vi "诊断标定3 - 副本.vi"(8 "CAN端口":u16(ring), 9 "设备索引号":u16(ring), 10 "CAN卡类型":u32(ring)=21) -> ()   [LabVIEW 2013] (continued)
                                n3186 = Reverse 1D Array(array=w4302) -> (reversed array=w4301:i32[])
                                n3187 = for {
                                N: w4297 -> [_]
                                tunnel: w4301 -> [w4319] mode=indexing
                                tunnel: [w4315] -> w4299 mode=indexing
                                n3188 = Equal To 0?(x=w4319) -> (x = 0?=w4318:bool)
                                n3189 = Select(t="无", s=w4318, f="故障") -> (s? t:f=w4315:string)
                                }
                                n3190 = Insert Into Array(array=w4300, new element=w4299) -> (w4298:string[])  [unwired: 1 in]
                              }
                              n3191 = call "详细故障分解.vi"("名称"=string[] ["自检异常(ee_cpu)", "存储空间满(ee_cpu)", "数据写入失败(ee_cpu)", "数据读取异常(ee_cpu)", "自检异常(ee_ext)", "存储空间满(ee_ext)", "数据写入失败(ee_ext)", "数据读取异常(ee_ext)", "自检异常(flash_ext)", "故障数据存储空间满(flash_ext)", "历史数据存储空间满(flash_ext)", "数据写入失败(flash_ext)", "数据读取失败(flash_ext)", "数据校验异常(flash_ext)", "自检异常(flash_cpu)", "存储空间满(flash_cpu)", "数据写入失败(flash_cpu)", "数据读取异常(flash_cpu)", "应用程序异常(cpu)", "应用程序下载异常(cpu)", "AD模块异常(cpu)", "RAM异常(cpu)", "CPU异常下电(cpu)"], "故障输入口"=w4292) -> ("输出数组"=w4290:string[][])  [unwired: 1 in, 2 out]
                              n3192 = local write "电池故障"(w4290) -> ()
                            }
                            frame 3 {
                              n3193 = for {
                                N: 5 -> [_]
                                tunnel: w4324 -> [w4341]
                                shift-right: [w4328] -> w4322
                                shift-left: string[] [] -> [w4330]
                                i -> [w4327]
                                w4335 = 8 ("索引")
                                w4339 = 2 ("y")
                                n3194 = Multiply(x=w4327, y=w4339) -> (x*y=w4340:i32)
                                n3195 = Array Subset(array=w4341, index=w4340, length=w4339) -> (w4338:u8[])
                                n3196 = Index Array(array=w4338) -> (element #1=w4337:u8, element #2=w4336:u8)  [unwired: 2 in]
                                n3197 = call "二进制解析-8.6.vi"("索引"=w4335, "数值"=w4337) -> ("低位子数组"=w4334:i32[])  [unwired: 1 in, 2 out]
                                n3198 = call "二进制解析-8.6.vi"("索引"=w4335, "数值"=w4336) -> ("低位子数组"=w4333:i32[])  [unwired: 1 in, 2 out]
                                n3199 = Insert Into Array(array=w4334, new element=w4333) -> (w4332:i32[])  [unwired: 1 in]
                                n3200 = Reverse 1D Array(array=w4332) -> (reversed array=w4331:i32[])
                                n3201 = for {
                                N: 6 -> [_]
                                tunnel: w4331 -> [w4346] mode=indexing
                                tunnel: [w4342] -> w4329 mode=indexing
                                n3202 = Equal To 0?(x=w4346) -> (x = 0?=w4345:bool)
                                n3203 = Select(t="无", s=w4345, f="故障") -> (s? t:f=w4342:string)
                                }
                                n3204 = Insert Into Array(array=w4330, new element=w4329) -> (w4328:string[])  [unwired: 1 in]
                              }
                              n3205 = call "详细故障分解.vi"("名称"=string[] ["初始化失败(CAN4)", "发送异常(CAN4)", "接收异常(CAN4)", "总线超时(CAN4)", "BUSOFF(CAN4)", "帧格式(CAN4)", "初始化异常(CAN0)", "发送异常(CAN0)", "接收异常(CAN0)", "总线超时(CAN0)", "BUSOFF(CAN0)", "帧格式(CAN0)", "初始化异常(CAN1)", "发送异常(CAN1)", "接收异常(CAN1)", "总线超时(CAN1)", "BUSOFF(CAN1)", "帧格式(CAN1)", "初始化失败(CAN2)", "发送异常(CAN2)", "接收异常(CAN2)", "总线超时(CAN2)", "BUSOFF(CAN2)", "帧格式(CAN2)", "初始化失败(CAN3)", "发送异常(CAN3)", "接收异常(CAN3)", "总线超时(CAN3)", "BUSOFF(CAN3)", "帧格式(CAN3)"], "故障输入口"=w4322) -> ("输出数组"=w4320:string[][])  [unwired: 1 in, 2 out]
                              n3206 = local write "电池故障"(w4320) -> ()
                            }
                            frame 4 {
                              n3207 = for {
                                N: 1 -> [_]
                                tunnel: w4351 -> [w4368]
                                shift-right: [w4355] -> w4349
                                shift-left: string[] [] -> [w4357]
                                i -> [w4354]
                                w4362 = 8 ("索引")
                                w4366 = 2 ("y")
                                n3208 = Multiply(x=w4354, y=w4366) -> (x*y=w4367:i32)
                                n3209 = Array Subset(array=w4368, index=w4367, length=w4366) -> (w4365:u8[])
                                n3210 = Index Array(array=w4365) -> (element #1=w4364:u8, element #2=w4363:u8)  [unwired: 2 in]
                                n3211 = call "二进制解析-8.6.vi"("索引"=w4362, "数值"=w4364) -> ("低位子数组"=w4361:i32[])  [unwired: 1 in, 2 out]
                                n3212 = call "二进制解析-8.6.vi"("索引"=w4362, "数值"=w4363) -> ("低位子数组"=w4360:i32[])  [unwired: 1 in, 2 out]
                                n3213 = Insert Into Array(array=w4361, new element=w4360) -> (w4359:i32[])  [unwired: 1 in]
                                n3214 = Reverse 1D Array(array=w4359) -> (reversed array=w4358:i32[])
                                n3215 = for {
                                N: 4 -> [_]
                                tunnel: w4358 -> [w4373] mode=indexing
                                tunnel: [w4369] -> w4356 mode=indexing
                                n3216 = Equal To 0?(x=w4373) -> (x = 0?=w4372:bool)
                                n3217 = Select(t="无", s=w4372, f="故障") -> (s? t:f=w4369:string)
                                }
                                n3218 = Insert Into Array(array=w4357, new element=w4356) -> (w4355:string[])  [unwired: 1 in]
                              }
                              n3219 = call "详细故障分解.vi"("名称"=string[] ["通讯协议版本不一致(soft)", "系统不同步(soft)", "软件版本不一致(soft)", "同硬件平台不兼容(soft)"], "故障输入口"=w4349) -> ("输出数组"=w4347:string[][])  [unwired: 1 in, 2 out]
                              n3220 = local write "电池故障"(w4347) -> ()
                            }
                            frame 5 {
                              n3221 = for {
                                N: 2 -> [_]
                                tunnel: w4378 -> [w4395]
                                shift-right: [w4382] -> w4376
                                shift-left: string[] [] -> [w4384]
                                i -> [w4381]
                                w4389 = 8 ("索引")
                                w4393 = 2 ("y")
                                n3222 = Multiply(x=w4381, y=w4393) -> (x*y=w4394:i32)
                                n3223 = Array Subset(array=w4395, index=w4394, length=w4393) -> (w4392:u8[])
                                n3224 = Index Array(array=w4392) -> (element #1=w4391:u8, element #2=w4390:u8)  [unwired: 2 in]
                                n3225 = call "二进制解析-8.6.vi"("索引"=w4389, "数值"=w4391) -> ("低位子数组"=w4388:i32[])  [unwired: 1 in, 2 out]
                                n3226 = call "二进制解析-8.6.vi"("索引"=w4389, "数值"=w4390) -> ("低位子数组"=w4387:i32[])  [unwired: 1 in, 2 out]
                                n3227 = Insert Into Array(array=w4388, new element=w4387) -> (w4386:i32[])  [unwired: 1 in]
                                n3228 = Reverse 1D Array(array=w4386) -> (reversed array=w4385:i32[])
                                n3229 = for {
                                N: 4 -> [_]
                                tunnel: w4385 -> [w4400] mode=indexing
                                tunnel: [w4396] -> w4383 mode=indexing
                                n3230 = Equal To 0?(x=w4400) -> (x = 0?=w4399:bool)
                                n3231 = Select(t="无", s=w4399, f="故障") -> (s? t:f=w4396:string)
                                }
                                n3232 = Insert Into Array(array=w4384, new element=w4383) -> (w4382:string[])  [unwired: 1 in]
                              }
                              n3233 = call "详细故障分解.vi"("名称"=string[] ["初始化失败(RS232)", "发送异常(RS232)", "接收异常(RS232)", "总线超时(RS232)", "初始化失败(RS485)", "发送异常(RS485)", "接收异常(RS485)", "总线超时(RS485)"], "故障输入口"=w4376) -> ("输出数组"=w4374:string[][])  [unwired: 1 in, 2 out]
                              n3234 = local write "电池故障"(w4374) -> ()
                            }
                            frame 6 {
                              n3235 = for {
                                N: 2 -> [_]
                                tunnel: w4405 -> [w4422]
                                shift-right: [w4409] -> w4403
                                shift-left: string[] [] -> [w4411]
                                i -> [w4408]
                                w4416 = 8 ("索引")
                                w4420 = 2 ("y")
                                n3236 = Multiply(x=w4408, y=w4420) -> (x*y=w4421:i32)
                                n3237 = Array Subset(array=w4422, index=w4421, length=w4420) -> (w4419:u8[])
                                n3238 = Index Array(array=w4419) -> (element #1=w4418:u8, element #2=w4417:u8)  [unwired: 2 in]
                                n3239 = call "二进制解析-8.6.vi"("索引"=w4416, "数值"=w4418) -> ("低位子数组"=w4415:i32[])  [unwired: 1 in, 2 out]
                                n3240 = call "二进制解析-8.6.vi"("索引"=w4416, "数值"=w4417) -> ("低位子数组"=w4414:i32[])  [unwired: 1 in, 2 out]
                                n3241 = Insert Into Array(array=w4415, new element=w4414) -> (w4413:i32[])  [unwired: 1 in]
                                n3242 = Reverse 1D Array(array=w4413) -> (reversed array=w4412:i32[])
                                n3243 = for {
                                N: 16 -> [_]
                                tunnel: w4412 -> [w4427] mode=indexing
                                tunnel: [w4423] -> w4410 mode=indexing
                                n3244 = Equal To 0?(x=w4427) -> (x = 0?=w4426:bool)
                                n3245 = Select(t="无", s=w4426, f="故障") -> (s? t:f=w4423:string)
                                }
                                n3246 = Insert Into Array(array=w4411, new element=w4410) -> (w4409:string[])  [unwired: 1 in]
                              }
                              n3247 = call "详细故障分解.vi"("名称"=string[] ["DI1对地短", "DI1对电源短", "DI2对地短", "DI2对电源短", "DI3对地短", "DI3对电源短", "DI4对地短", "DI4对电源短", "DI5对地短", "DI5对电源短", "DI6对地短", "DI6对电源短", "DI7对地短", "DI7对电源短", "DI8对地短", "DI8对电源短", "DO1对地短", "DO1对电源短", "DO2对地短", "DO2对电源短", "DO3对地短", "DO3对电源短", "DO4对地短", "DO4对电源短", "DO5对地短", "DO5对电源短", "DO6对地短", "DO6对电源短", "DO7对地短", "DO7对电源短", "DO8对地短", "DO8对电源短"], "故障输入口"=w4403) -> ("输出数组"=w4401:string[][])  [unwired: 1 in, 2 out]
                              n3248 = local write "电池故障"(w4401) -> ()
                            }
                            frame 7 {
                              n3249 = for {
                                N: 2 -> [_]
                                tunnel: w4432 -> [w4449]
                                shift-right: [w4436] -> w4430
                                shift-left: string[] [] -> [w4438]
                                i -> [w4434]
                                w4443 = 8 ("索引")
                                w4447 = 2 ("y")
                                n3250 = Multiply(x=w4434, y=w4447) -> (x*y=w4448:i32)
                                n3251 = Array Subset(array=w4449, index=w4448, length=w4447) -> (w4446:u8[])
                                n3252 = Index Array(array=w4446) -> (element #1=w4445:u8, element #2=w4444:u8)  [unwired: 2 in]
                                n3253 = call "二进制解析-8.6.vi"("索引"=w4443, "数值"=w4445) -> ("低位子数组"=w4442:i32[])  [unwired: 1 in, 2 out]
                                n3254 = call "二进制解析-8.6.vi"("索引"=w4443, "数值"=w4444) -> ("低位子数组"=w4441:i32[])  [unwired: 1 in, 2 out]
                                n3255 = Insert Into Array(array=w4442, new element=w4441) -> (w4440:i32[])  [unwired: 1 in]
                                n3256 = case shown="1" w4434 {
                                tunnel: [4 6] -> w4435
                                frame 0, Default {
                                }
                                frame 1 {
                                }
                                }
                                n3257 = Reverse 1D Array(array=w4440) -> (reversed array=w4439:i32[])
                                n3258 = for {
                                N: w4435 -> [_]
                                tunnel: w4439 -> [w4456] mode=indexing
                                tunnel: [w4452] -> w4437 mode=indexing
                                n3259 = Equal To 0?(x=w4456) -> (x = 0?=w4455:bool)
                                n3260 = Select(t="无", s=w4455, f="故障") -> (s? t:f=w4452:string)
                                }
                                n3261 = Insert Into Array(array=w4438, new element=w4437) -> (w4436:string[])  [unwired: 1 in]
                              }
                              n3262 = call "详细故障分解.vi"("名称"=string[] ["超时(pre-chg)", "后端开路(pre-chg)", "后端短路(pre-chg)", "预充电回路断开(pre-chg)", "正级继电器驱动故障(relay_driver)", "负级继电器驱动故障(relay_driver)", "预充电继电器驱动故障(relay_driver)", "充电继电器驱动故障(relay_driver)", "风机继电器驱动故障(relay_driver)", "加热继电器驱动故障(relay_driver)"], "故障输入口"=w4430) -> ("输出数组"=w4428:string[][])  [unwired: 1 in, 2 out]
                              n3263 = local write "电池故障"(w4428) -> ()
                            }
                          }
                        }
                        frame True {
                          n3264 = Index Array(array=w4460, index #1=0 ("索引"), index #2=1 ("索引")) -> (element #1=w4463:u8, element #2=w4464:u8)
                          n3265 = Join Numbers(hi=w4463, lo=w4464) -> ((hi.lo)=w4462:u16)
                          n3266 = Number To Hexadecimal String(2:w4462) -> (0:w4461:string)  [unwired: 1 out]
                          n3267 = Concatenate Strings("读取错误，代码： " ("字符串"), "0x" ("字符串"), w4461) -> (w4459:string)
                          n3268 = One Button Dialog(message=w4459, button name ("OK")="是" ("按钮名称（“确定”）")) -> ()  [unwired: 1 out]
                        }
                      }
                      n3269 = local write "消除"(FALSE ("消除")) -> ()
                      n3270 = global write "EV05全局变量1.vi" "流控帧 2"(FALSE ("流控帧 2")) -> ()
                      n3271 = local write "控制1"(FALSE ("控制1")) -> ()
                      n3272 = global write "EV05全局变量1.vi" "写入超时"(TRUE ("写入超时")) -> ()
                    }
                  }
                }
              }
            }
          }
        }
      }
      frame Error {
      }
    }
  }
  n3273 = local write "二维码"(w1) -> ()
  n3274 = call <vilib>:"Close Config Data.vi"("error in (no error)"=w9, "refnum"=w10) -> ("error out"=w2:errorcluster)  [unwired: 8 in, 1 out]
  n3275 = case shown="无错误" w11 {
    tunnel: w2 -> [_ _]
    frame No Error {
      n3276 = case shown="\"全部读取\"" "全部写入" {
        frame "假", Default {
          n3277 = local write "强制终止读写标记"(FALSE ("强制终止读写标记")) -> ()
        }
        frame "单个写入" {
          n3278 = local read "主从选择"() -> (w4476:enum32{"主板", "从板"})
          n3279 = case shown="\"主板\", 默认" w4476 {
            tunnel: [w4487 w4502] -> w4473
            tunnel: [0.0 w4500] -> w4477
            tunnel: [_ w4501] -> w4475
            tunnel: [w4485 _] -> w4474
            frame "主板", Default {
              n3280 = stacked-sequence {
                tunnel: [_ w4499] -> w4485
                frame #0 {
                  n3281 = control-ref of="高压参数"() -> (w4490:refnum<vi>)
                  n3282 = control-ref of="电池信息"() -> (w4491:refnum<vi>)
                  n3283 = control-ref of="一级故障"() -> (w4497:refnum<vi>)
                  n3284 = control-ref of="一级故障 2"() -> (w4495:refnum<vi>)
                  n3285 = control-ref of="一级故障 3"() -> (w4494:refnum<vi>)
                  n3286 = control-ref of="加热控制参数"() -> (w4493:refnum<vi>)
                  n3287 = control-ref of="充电控制参数"() -> (w4492:refnum<vi>)
                  n3288 = control-ref of="项目信息"() -> (w4496:refnum<vi>)
                  n3289 = control-ref of="项目信息2"() -> (w4498:refnum<vi>)
                  n3290 = local read "主板数据"() -> (w4488:T4)
                  n3291 = Bundle(cluster=w4488, "项目信息"=w4496, "一级故障 4"=w4498, "一级故障"=w4497, "一级故障 2"=w4495, "一级故障 3"=w4494, "加热控制参数"=w4493, "充电控制参数"=w4492, "高压参数"=w4490, "电池信息"=w4491) -> (w4489:T4)
                  n3292 = local write "主板数据"(w4489) -> ()
                }
                frame #1 {
                  n3293 = control-ref of="主板数据"() -> (w4499:refnum<vi>)
                }
              }
              n3294 = local read "主板选项"() -> (w4487:string)
            }
            frame "从板" {
              n3295 = stacked-sequence {
                tunnel: [_ w4513] -> w4501
                frame #0 {
                  n3296 = control-ref of="从板号"() -> (w4512:refnum<vi>)
                  n3297 = control-ref of="项目信息 2"() -> (w4511:refnum<vi>)
                  n3298 = control-ref of="均衡参数"() -> (w4506:refnum<vi>)
                  n3299 = control-ref of="加热控制参数"() -> (w4510:refnum<vi>)
                  n3300 = control-ref of="一级故障(从板)"() -> (w4509:refnum<vi>)
                  n3301 = control-ref of="二级故障(从板)"() -> (w4508:refnum<vi>)
                  n3302 = control-ref of="三级故障(从板)"() -> (w4507:refnum<vi>)
                  n3303 = control-ref of="电池组信息"() -> (w4503:refnum<vi>)
                  n3304 = local read "从板信息"() -> (w4504:T2)
                  n3305 = Bundle(cluster=w4504, "从板号"=w4512, "项目信息 2"=w4511, "加热控制参数"=w4510, "一级故障(从板)"=w4509, "二级故障(从板)"=w4508, "三级故障(从板)"=w4507, "电池组信息(从板)"=w4503, "均衡参数"=w4506) -> (w4505:T2)
                  n3306 = local write "从板信息"(w4505) -> ()
                }
                frame #1 {
                  n3307 = control-ref of="从板信息"() -> (w4513:refnum<vi>)
                }
              }
              n3308 = local read "从板选项"() -> (w4502:string)
              n3309 = local read "从板号"() -> (w4500:u8)
            }
          }
          n3310 = local read "从板个数"() -> (w4478:dbl)
          n3311 = local read "快换"() -> (w4479:bool)
          n3312 = call "输入数据解析.vi"("单个参数补充"=w4478, "从板号"=w4477, "主板引用"=w4474, "从板引用"=w4475, "主板选项"=w4473, "枚举"=w4476, "快换"=w4479) -> ("输出数组"=w4483:dbl[][], "数组长度"=w4482:dbl[], "循环次数"=w4472:i32, "命令"=w4481:u32, "名称"=w4471:string[], "命令序号"=w4480:u32[])  [unwired: 2 in, 1 out]
          n3313 = for {
            N: w4472 -> [w4519]
            tunnel: w4483 -> [w4529]
            tunnel: w4482 -> [w4528]
            tunnel: w4481 -> [w4527]
            tunnel: w4480 -> [w4526]
            tunnel: w4477 -> [w4517]
            tunnel: w4473 -> [w4525]
            tunnel: w4471 -> [w4521]
            tunnel: [w4514] -> w4470
            i -> [w4520]
            n3314 = Index Array(array=w4529, index (row)=w4520) -> (element=w4524:dbl[])  [unwired: 1 in]
            n3315 = Index Array(array=w4528, index=w4520) -> (element=w4523:dbl)
            n3316 = Index Array(array=w4521, index=w4520) -> (element=w4518:string)
            n3317 = case shown="\"假\", 默认" w4518 {
              tunnel: [w4531 w4532] -> w4516
              tunnel: w4517 -> [w4531 _]
              tunnel: [TRUE ("确定") w4533] -> w4515
              frame "假", Default {
              }
              frame "从板号" {
                n3318 = call "请输入当前从板板号"() -> ("当前从板板号"=w4532:dbl, "确定"=w4533:bool)  [unwired: 17 in, 1 out]
                n3319 = local write "当前从板板号"(w4532) -> ()
              }
            }
            n3320 = Index Array(array=w4526, index=w4520) -> (element=w4522:u32)
            n3321 = global write "全局 1.vi" "名称"(w4518) -> ()
            n3322 = case shown="真" w4515 {
              tunnel: w4527 -> [_ w4543]
              tunnel: w4525 -> [_ w4542]
              tunnel: w4524 -> [_ w4541]
              tunnel: w4523 -> [_ w4540]
              tunnel: w4522 -> [_ w4539]
              tunnel: w4520 -> [_ w4538]
              tunnel: w4518 -> [_ w4537]
              tunnel: w4519 -> [_ w4536]
              tunnel: w4516 -> [_ w4535]
              tunnel: [_ w4534] -> w4514
              frame False {
                n3323 = call <vilib>:"Unset Busy.vi"() -> ()  [unwired: 11 in, 1 out]
              }
              frame True {
                n3324 = stacked-sequence {
                  seq-local: [_ _ _ w4571 _ _] -> [_ _ _ _ w4580 _]
                  tunnel: w4541 -> [_ _ w4556 _ _ _]
                  tunnel: w4540 -> [_ _ w4555 _ _ _]
                  tunnel: w4543 -> [_ _ w4549 _ _ _]
                  tunnel: w4539 -> [_ _ w4547 _ _ _]
                  tunnel: w4542 -> [_ _ _ _ _ _]
                  tunnel: w4538 -> [_ _ _ _ _ w4591]
                  tunnel: w4537 -> [_ _ _ _ w4579 _]
                  tunnel: w4536 -> [_ _ _ _ _ w4592]
                  tunnel: w4535 -> [_ _ w4548 _ _ _]
                  tunnel: [_ _ _ _ _ w4589] -> w4534
                  frame #0 {
                    w4545 = FALSE ("流控帧")
                    w4544 = TRUE ("流控帧 2")
                    n3325 = call <vilib>:"Set Busy.vi"("disable click? (T)"=w4545) -> ()  [unwired: 3 in, 8 out]
                    n3326 = global write "EV05全局变量1.vi" "读取超时"(w4545) -> ()
                    n3327 = global write "EV05全局变量1.vi" "流控帧"(w4545) -> ()
                    n3328 = local write "消除"(w4544) -> ()
                    n3329 = local write "控制1"(w4544) -> ()
                    n3330 = global write "EV05全局变量1.vi" "流控帧 2"(w4544) -> ()
                    n3331 = local write "写?"(w4544) -> ()
                  }
                  frame #1 {
                    n3332 = Wait Until Next ms Multiple(millisecond multiple=u32 50 ("毫秒倍数")) -> ()  [unwired: 1 out]
                  }
                  frame #2 {
                    n3333 = local read "设备索引号"() -> (w4551:u16)
                    n3334 = local read "CAN卡类型"() -> (w4552:u32)
                    n3335 = Increment(x=w4555) -> (x+1=w4554:dbl)
                    n3336 = local read "CAN端口"() -> (w4550:u16)
                    n3337 = local write "命令"(w4549) -> ()
                    n3338 = local write "命令序号"(w4547) -> ()
                    n3339 = Reshape Array(w4556, w4554) -> (w4553:dbl[])
                    n3340 = stacked-sequence {
                      tunnel: w4553 -> [_ w4570]
                      tunnel: w4552 -> [w4559 w4569]
                      tunnel: w4551 -> [w4558 w4568]
                      tunnel: w4550 -> [w4557 w4567]
                      tunnel: w4549 -> [_ w4566]
                      tunnel: w4548 -> [_ w4565]
                      tunnel: w4547 -> [_ w4564]
                      frame #0 {
                        n3341 = disable-structure shown="禁用" {
                          disable-tunnel: w4559 -> [w4562 _]
                          disable-tunnel: w4558 -> [w4561 _]
                          disable-tunnel: w4557 -> [w4560 _]
                          frame Disabled {
                            n3342 = dll-call lib="PTH1mabs FBluewave New EnergySVN_WorkBMS_Monitor_Bnet01trunk参数设置data\nkerneldlls\nusbcan.dll" fn="VCI_ClearBuffer"("DeviceType"=w4562, "DeviceInd"=w4561, "CANInd"=w4560) -> (error out=w4563:errorcluster)  [unwired: 4 in, 4 out]
                            n3343 = call <vilib>:"Clear Errors.vi"("error in (no error)"=w4563) -> ()  [unwired: 6 in, 1 out]
                          }
                          frame Enabled {
                          }
                        }
                      }
                      frame #1 {
                        n3344 = call "多帧发送机制(EV05).vi"("can卡类型"=w4569, "设备索引号"=w4568, "CAN端口"=w4567, "命令"=w4566, "板号"=w4565, "命令序号"=w4564, "输入数据"=w4570) -> ()  [unwired: 1 in, 12 out]
                      }
                    }
                  }
                  frame #3 {
                    n3345 = while {
                      tunnel: [w4573] -> w4571
                      i -> [w4577]
                      stop <- w4574 stop-if-true
                      n3346 = local read "强制终止读写标记"() -> (w4572:bool)
                      n3347 = global read "EV05全局变量1.vi" "读取超时"() -> (w4573:bool)
                      n3348 = Greater Or Equal?(x=w4577, y=30) -> (x >= y?=w4575:bool)
                      n3349 = Wait Until Next ms Multiple(millisecond multiple=u32 100 ("毫秒倍数")) -> ()  [unwired: 1 out]
                      n3350 = Compound Arithmetic op=OR(w4572, w4573, w4575) -> (w4574:bool)
                    }
                  }
                  frame #4 {
                    n3351 = case shown="假" w4580 {
                      tunnel: w4579 -> [w4581 w4587]
                      frame False {
                        n3352 = control-ref of="结果"() -> (w4585:refnum<vi>)
                        n3353 = Concatenate Strings(w4581, "       写入失败" ("字符串")) -> (w4584:string)
                        n3354 = Build Array(w4584) -> (w4583:string[])
                        n3355 = call "表格编辑.vi"("新元素/子数组"=w4583, "活动单元格:单元格背景色"=u32 16740749, "MCListbox引用句柄"=w4585) -> ()  [unwired: 9 out]
                      }
                      frame True {
                        n3356 = case shown="\"从板号\"" w4587 {
                          frame "假", Default {
                          }
                          frame "从板号" {
                            n3357 = local read "从板号"() -> (w4588:u8)
                            n3358 = local write "当前从板板号"(w4588) -> ()
                          }
                        }
                      }
                    }
                    n3359 = call <vilib>:"Unset Busy.vi"() -> ()  [unwired: 2 in, 10 out]
                  }
                  frame #5 {
                    n3360 = Increment(x=w4591) -> (x+1=w4590:i32)
                    n3361 = Equal?(x=w4592, y=w4590) -> (x = y?=w4589:bool)
                    n3362 = case shown="真" w4589 {
                      frame False {
                      }
                      frame True {
                        n3363 = control-ref of="结果"() -> (w4596:refnum<vi>)
                        n3364 = Concatenate Strings("写入完成" ("字符串")) -> (w4595:string)
                        n3365 = Build Array(w4595) -> (w4594:string[])
                        n3366 = call "表格编辑.vi"("新元素/子数组"=w4594, "活动单元格:单元格背景色"=u32 21937, "MCListbox引用句柄"=w4596) -> ()  [unwired: 9 out]
                      }
                    }
                  }
                }
              }
            }
          }
          n3367 = stacked-sequence {
            tunnel: w4470 -> [_]
            frame #0 {
              n3368 = call <vilib>:"Unset Busy.vi"() -> ()  [unwired: 2 in, 10 out]
              n3369 = local write "强制终止读写标记"(FALSE ("强制停止")) -> ()
            }
          }
        }
        frame "全部写入" {
          n3370 = local read "主从选择"() -> (w4604:enum32{"主板", "从板"})
          n3371 = case shown="\"主板\", 默认" w4604 {
            tunnel: [string[] ["项目信息", "一级故障阀值", "二级故障阀值", "三级故障阀值", "加热控制参数", "充电控制参数", "电池信息", "二维码"] string[] ["从板信息", "一级故障阀值", "二级故障阀值", "三级故障阀值", "均衡参数"]] -> w4601
            tunnel: [0.0 ("从板号") w4781] -> w4605
            tunnel: [w4766 _] -> w4603
            tunnel: [_ w4782] -> w4602
            frame "主板", Default {
              n3372 = stacked-sequence {
                tunnel: [_ w4780] -> w4766
                frame #0 {
                  n3373 = control-ref of="电池信息"() -> (w4772:refnum<vi>)
                  n3374 = control-ref of="高压参数"() -> (w4771:refnum<vi>)
                  n3375 = control-ref of="一级故障"() -> (w4774:refnum<vi>)
                  n3376 = control-ref of="一级故障 2"() -> (w4776:refnum<vi>)
                  n3377 = control-ref of="一级故障 3"() -> (w4777:refnum<vi>)
                  n3378 = control-ref of="加热控制参数"() -> (w4778:refnum<vi>)
                  n3379 = control-ref of="充电控制参数"() -> (w4779:refnum<vi>)
                  n3380 = control-ref of="项目信息"() -> (w4775:refnum<vi>)
                  n3381 = control-ref of="项目信息2"() -> (w4773:refnum<vi>)
                  n3382 = local read "主板数据"() -> (w4770:T4)
                  n3383 = Bundle(cluster=w4770, "项目信息"=w4775, "一级故障 4"=w4773, "一级故障"=w4774, "一级故障 2"=w4776, "一级故障 3"=w4777, "加热控制参数"=w4778, "充电控制参数"=w4779, "高压参数"=w4771, "电池信息"=w4772) -> (w4769:T4)
                  n3384 = local write "主板数据"(w4769) -> ()
                }
                frame #1 {
                  n3385 = control-ref of="主板数据"() -> (w4780:refnum<vi>)
                }
              }
              n3386 = local write "失败?"(FALSE ("失败?")) -> ()
            }
            frame "从板" {
              (unwired) "均衡参数"
              n3387 = stacked-sequence {
                tunnel: [_ w4794] -> w4782
                frame #0 {
                  n3388 = control-ref of="从板号"() -> (w4788:refnum<vi>)
                  n3389 = control-ref of="项目信息 2"() -> (w4789:refnum<vi>)
                  n3390 = control-ref of="均衡参数"() -> (w4786:refnum<vi>)
                  n3391 = control-ref of="加热控制参数"() -> (w4790:refnum<vi>)
                  n3392 = control-ref of="一级故障(从板)"() -> (w4791:refnum<vi>)
                  n3393 = control-ref of="二级故障(从板)"() -> (w4792:refnum<vi>)
                  n3394 = control-ref of="三级故障(从板)"() -> (w4793:refnum<vi>)
                  n3395 = control-ref of="电池组信息"() -> (w4787:refnum<vi>)
                  n3396 = local read "从板信息"() -> (w4785:T2)
                  n3397 = Bundle(cluster=w4785, "从板号"=w4788, "项目信息 2"=w4789, "加热控制参数"=w4790, "一级故障(从板)"=w4791, "二级故障(从板)"=w4792, "三级故障(从板)"=w4793, "电池组信息(从板)"=w4787, "均衡参数"=w4786) -> (w4784:T2)
                  n3398 = local write "从板信息"(w4784) -> ()
                }
                frame #1 {
                  n3399 = control-ref of="从板信息"() -> (w4794:refnum<vi>)
                }
              }
              n3400 = local read "从板号"() -> (w4781:u8)
            }
          }
          n3401 = Array Size(array=w4601) -> (size(s)=w4600:i32)
          n3402 = while {
            tunnel: w4601 -> [w4639] mode=indexing
            tunnel: w4604 -> [w4643]
            tunnel: w4605 -> [w4646]
            tunnel: w4603 -> [w4645]
            tunnel: w4602 -> [w4644]
            tunnel: w4600 -> [w4637]
            tunnel: [w4633] -> w4599
            i -> [w4638]
            stop <- w4634 stop-if-true
            n3403 = local read "二维码"() -> (w4632:string)
            n3404 = Increment(x=w4638) -> (x+1=w4636:i32)
            n3405 = local read "从板个数"() -> (w4651:dbl)
            n3406 = local read "快换"() -> (w4642:bool)
            n3407 = Less Or Equal?(x=w4637, y=w4636) -> (x <= y?=w4633:bool)
            n3408 = call "输入数据解析.vi"("单个参数补充"=w4651, "从板号"=w4646, "主板二维码"=w4632, "主板引用"=w4645, "从板引用"=w4644, "主板选项"=w4639, "枚举"=w4643, "快换"=w4642) -> ("输出数组"=w4650:dbl[][], "数组长度"=w4649:dbl[], "循环次数"=w4641:i32, "命令"=w4648:u32, "名称"=w4640:string[], "命令序号"=w4647:u32[])  [unwired: 1 in, 1 out]
            n3409 = case shown="\"主板\", 默认" w4643 {
              tunnel: w4638 -> [w4653 w4667]
              frame "主板", Default {
                n3410 = case shown="6" w4653 {
                  tunnel: [T8."项目信息" ("主从板") T8."一级故障阀值" ("主从板") T8."二级故障阀值" ("主从板") T8."三级故障阀值" ("主从板") T8."控制参数" ("主从板") T8."电池信息" ("主从板")] -> w4652
                  frame 0, Default {
                    n3411 = local write "1"(TRUE ("1")) -> ()
                  }
                  frame 1 {
                    n3412 = local write "1 2"(TRUE ("1 2")) -> ()
                  }
                  frame 2 {
                    n3413 = local write "1 3"(TRUE ("1 3")) -> ()
                  }
                  frame 3 {
                    n3414 = local write "1 4"(TRUE ("1 4")) -> ()
                  }
                  frame 4, 5 {
                    n3415 = local write "1 5"(TRUE ("1 5")) -> ()
                  }
                  frame 6 {
                    n3416 = local write "1 11"(TRUE ("1 11")) -> ()
                  }
                }
                n3417 = local write "主板2"(w4652) -> ()
              }
              frame "从板" {
                n3418 = case shown="1" w4667 {
                  tunnel: [T21."从板信息" ("等级 2") T21."从板信息" ("等级 2") T21."一级故障阀值" ("等级 2") T21."二级故障阀值" ("等级 2") T21."三级故障阀值" ("等级 2") T21."快换参数" ("等级 2") T14."均衡参数" ("等级 2")] -> w4666
                  frame 99, Default {
                    n3419 = local write "1 6"(TRUE ("1 6")) -> ()
                  }
                  frame 0 {
                    n3420 = local write "1 6"(TRUE ("1 6")) -> ()
                  }
                  frame 1 {
                    n3421 = local write "1 7"(TRUE ("1 7")) -> ()
                  }
                  frame 2 {
                    n3422 = local write "1 8"(TRUE ("1 8")) -> ()
                  }
                  frame 3 {
                    n3423 = local write "1 9"(TRUE ("1 9")) -> ()
                  }
                  frame 4 {
                    n3424 = local write "1 10"(TRUE ("1 10")) -> ()
                  }
                  frame 5 {
                    n3425 = local write "1 12"(TRUE ("1 10")) -> ()
                  }
                }
                n3426 = local write "等级 2"(w4666) -> ()
              }
            }
            n3427 = for {
              N: w4641 -> [w4684]
              tunnel: w4650 -> [w4694]
              tunnel: w4649 -> [w4693]
              tunnel: w4648 -> [w4692]
              tunnel: w4647 -> [w4690]
              tunnel: w4646 -> [w4691]
              tunnel: w4640 -> [w4687]
              tunnel: w4633 -> [w4682]
              i -> [w4683]
              n3428 = Index Array(array=w4694, index (row)=w4683) -> (element=w4689:dbl[])  [unwired: 1 in]
              n3429 = Index Array(array=w4693, index=w4683) -> (element=w4688:dbl)
              n3430 = Index Array(array=w4687, index=w4683) -> (element=w4685:string)
              n3431 = Index Array(array=w4690, index=w4683) -> (element=w4686:u32)
              n3432 = while {
                tunnel: w4692 -> [w4704]
                tunnel: w4691 -> [w4703]
                tunnel: w4689 -> [w4702]
                tunnel: w4688 -> [w4701]
                tunnel: w4686 -> [w4700]
                tunnel: w4685 -> [w4699]
                tunnel: w4684 -> [w4698]
                tunnel: w4683 -> [w4697]
                tunnel: w4682 -> [w4696]
                stop <- w4695 stop-if-true
                n3433 = stacked-sequence {
                  seq-local: [_ _ _ w4727 _ _] -> [_ _ _ _ w4736 _]
                  tunnel: w4702 -> [_ _ w4715 _ _ _]
                  tunnel: w4701 -> [_ _ w4714 _ _ _]
                  tunnel: w4704 -> [_ _ w4709 _ _ _]
                  tunnel: w4703 -> [_ _ w4712 _ _ _]
                  tunnel: w4700 -> [_ _ w4710 _ _ _]
                  tunnel: w4699 -> [_ _ w4708 _ w4737 _]
                  tunnel: w4698 -> [_ _ _ _ _ w4759]
                  tunnel: w4697 -> [_ _ _ _ _ w4758]
                  tunnel: w4696 -> [_ _ _ _ _ w4756]
                  tunnel: [_ _ _ _ w4735 _] -> w4695
                  frame #0 {
                    w4706 = FALSE ("流控帧")
                    w4705 = TRUE ("流控帧 2")
                    n3434 = call <vilib>:"Set Busy.vi"("disable click? (T)"=w4706) -> ()  [unwired: 3 in, 8 out]
                    n3435 = global write "EV05全局变量1.vi" "读取超时"(w4706) -> ()
                    n3436 = global write "EV05全局变量1.vi" "流控帧"(w4706) -> ()
                    n3437 = local write "消除"(w4705) -> ()
                    n3438 = local write "控制1"(w4705) -> ()
                    n3439 = global write "EV05全局变量1.vi" "流控帧 2"(w4705) -> ()
                    n3440 = local write "写?"(w4705) -> ()
                  }
                  frame #1 {
                    n3441 = Wait Until Next ms Multiple(millisecond multiple=u32 50 ("毫秒倍数")) -> ()  [unwired: 1 out]
                  }
                  frame #2 {
                    n3442 = global write "全局 1.vi" "名称"(w4708) -> ()
                    n3443 = local write "命令序号"(w4710) -> ()
                    n3444 = local write "命令"(w4709) -> ()
                    n3445 = local read "设备索引号"() -> (w4717:u16)
                    n3446 = local read "CAN卡类型"() -> (w4718:u32)
                    n3447 = Increment(x=w4714) -> (x+1=w4711:dbl)
                    n3448 = local read "CAN端口"() -> (w4716:u16)
                    n3449 = Reshape Array(w4715, w4711) -> (w4713:dbl[])
                    n3450 = stacked-sequence {
                      tunnel: w4718 -> [_ w4726]
                      tunnel: w4717 -> [_ w4725]
                      tunnel: w4716 -> [_ w4724]
                      tunnel: w4713 -> [_ w4723]
                      tunnel: w4712 -> [_ w4722]
                      tunnel: w4710 -> [_ w4721]
                      tunnel: w4709 -> [_ w4720]
                      frame #0 {
                      }
                      frame #1 {
                        n3451 = call "多帧发送机制(EV05).vi"("can卡类型"=w4726, "设备索引号"=w4725, "CAN端口"=w4724, "命令"=w4720, "板号"=w4722, "命令序号"=w4721, "输入数据"=w4723) -> ("错误输出"=w4719:errorcluster)  [unwired: 1 in, 11 out]
                        n3452 = call <vilib>:"Clear Errors.vi"("error in (no error)"=w4719) -> ()  [unwired: 6 in, 1 out]
                      }
                    }
                  }
                  frame #3 {
                    n3453 = while {
                      tunnel: [w4729] -> w4727
                      i -> [w4734]
                      stop <- w4731 stop-if-true
                      n3454 = local read "强制终止读写标记"() -> (w4728:bool)
                      n3455 = global read "EV05全局变量1.vi" "读取超时"() -> (w4729:bool)
                      n3456 = Greater Or Equal?(x=w4734, y=30) -> (x >= y?=w4732:bool)
                      n3457 = Wait Until Next ms Multiple(millisecond multiple=u32 100 ("毫秒倍数")) -> ()  [unwired: 1 out]
                      n3458 = Compound Arithmetic op=OR(w4728, w4729, w4732) -> (w4731:bool)
                    }
                  }
                  frame #4 {
                    n3459 = case shown="假" w4736 {
                      tunnel: w4737 -> [w4743 _]
                      tunnel: [w4738 TRUE] -> w4735
                      frame False {
                        n3460 = local read "重试次数"() -> (w4742:u8)
                        n3461 = Increment(x=w4742) -> (x+1=w4741:u8)
                        n3462 = Greater Or Equal?(x=w4741, y=u8 4) -> (x >= y?=w4739:bool)
                        n3463 = local write "重试次数"(w4741) -> ()
                        n3464 = case shown="真" w4739 {
                          tunnel: w4743 -> [w4746 _]
                          tunnel: [TRUE FALSE] -> w4738
                          frame False {
                            n3465 = control-ref of="结果"() -> (w4750:refnum<vi>)
                            n3466 = local write "失败?"(TRUE ("失败?")) -> ()
                            n3467 = Concatenate Strings(w4746, "       写入失败" ("字符串")) -> (w4749:string)
                            n3468 = Build Array(w4749) -> (w4748:string[])
                            n3469 = call "表格编辑.vi"("新元素/子数组"=w4748, "活动单元格:单元格背景色"=u32 16740749, "MCListbox引用句柄"=w4750) -> ()  [unwired: 9 out]
                          }
                          frame True {
                          }
                        }
                      }
                      frame True {
                      }
                    }
                  }
                  frame #5 {
                    n3470 = Increment(x=w4758) -> (x+1=w4754:i32)
                    n3471 = Equal?(x=w4759, y=w4754) -> (x = y?=w4757:bool)
                    n3472 = And(x=w4756, y=w4757) -> (x .and. y?=w4755:bool)
                    n3473 = case shown="真" w4755 {
                      frame False {
                      }
                      frame True {
                        n3474 = Concatenate Strings("写入完成" ("字符串")) -> (w4762:string)
                        n3475 = control-ref of="结果"() -> (w4763:refnum<vi>)
                        n3476 = Build Array(w4762) -> (w4761:string[])
                        n3477 = call "表格编辑.vi"("新元素/子数组"=w4761, "活动单元格:单元格背景色"=u32 21937, "MCListbox引用句柄"=w4763) -> ()  [unwired: 9 out]
                      }
                    }
                  }
                }
              }
            }
            n3478 = local read "强制终止读写标记"() -> (w4635:bool)
            n3479 = Or(x=w4633, y=w4635) -> (x .or. y?=w4634:bool)
          }
          n3480 = stacked-sequence {
            tunnel: [_ w4618 _ _] -> _
            tunnel: w4599 -> [_ _ _ _]
            frame #0 {
              n3481 = local read "失败?"() -> (w4609:bool)
              n3482 = Select(t="FAIL" ("key"), s=w4609, f="PASS" ("key")) -> (s? t:f=w4608:string)
              n3483 = call <vilib>:"Open Config Data.vi"("error in (no error)"=errorcluster {"status"=FALSE, "code"=0, "source"=""}, "configuration file path"=path "D:/BlueWay/configresult.ini") -> ("error out"=w4615:errorcluster, "refnum"=w4611:T19)  [unwired: 7 in, 1 out]
              n3484 = call-poly <vilib>:"Write Key.vi"("section"="BCURESULT", "error in (no error)"=w4615, "value"=w4608, "key"="BCURESULT", "refnum"=w4611) -> ("error out"=w4616:errorcluster, "refnum out"=w4612:T19)  [unwired: 4 in, 1 out]
              n3485 = call <vilib>:"Close Config Data.vi"("error in (no error)"=w4616, "refnum"=w4612) -> ()  [unwired: 8 in, 2 out]
            }
            frame #1 {
              w4625 = u8 0 items=["Normal", "Listen Only"] ("工作方式")
              w4624 = u8 1 items=["Dual Filter", "Single Filter"] ("滤波方式")
              n3486 = local read "设备索引号"() -> (w4620:u16)
              n3487 = local read "CAN卡类型"() -> (w4619:u32)
              n3488 = local read "CAN端口"() -> (w4621:u16)
              n3489 = call "CAN_Init-8.6.vi"("CAN卡类型"=w4619, "设备索引号"=w4620, "CAN端口"=w4621, "操作类型"=enum16{"初始化CAN", "关闭CAN"}."关闭CAN", "滤波方式"=w4624, "Accept Code"=u32 3221225472, "簇"=T23 {"打开CAN"=FALSE, "初始化CAN"=FALSE, "开始CAN"=FALSE, "重启"=TRUE, "关闭CAN"=TRUE}, "Mask Code"=u32 1073741823 ("Accept Code"), "工作方式"=w4625, "是否滤波"=TRUE, "滤波选择"=T22 {"fiter_mode"=1, "fiter_endid"=402653184, "fiter_startid"=419430399}) -> ("error out"=w4618:errorcluster)  [unwired: 3 in, 5 out]
            }
            frame #2 {
              n3490 = Quit LabVIEW(quit? (T)=TRUE ("退出？(T)")) -> ()
            }
            frame #3 {
              n3491 = local write "停止"(TRUE ("停止")) -> ()
            }
          }
          "失败?" <- FALSE
        }
        frame "单个读取" {
          n3492 = stacked-sequence {
            tunnel: [w4797] -> w4795
            frame #0 {
              n3493 = local read "主从选择"() -> (w4798:enum32{"主板", "从板"})
              n3494 = case shown="\"主板\", 默认" w4798 {
                tunnel: [w4811 w4891] -> w4800
                tunnel: [w4810 w4892] -> w4805
                tunnel: [0 ("从板号") w4888] -> w4804
                tunnel: [0 ("板号") u8 0 ("板号")] -> w4803
                tunnel: [w4806 w4887] -> w4801
                frame "主板", Default {
                  n3495 = local read "主板选项"() -> (w4807:string)
                  n3496 = case shown="\"SOC过低(3)\", \"SOC过高(3)\", \"SOH过低(3)\", \"充电电流过高(3)\", \"单体电压过低(3)\", \"单体电压过高(3)\", \"单组电压不均衡(3)\", \"单组温度不均衡(3)\", \"放电电流过高(3)\", \"极柱温度过高(3)\", \"内阻过大(3)\", \"三级故障阀值\", \"温度过低(3)\", \"温度过高(3)\", \"整组电压不均衡(3)\", \"整组温度不均衡(3)\", \"总电压过低(3)\", \"总电压过高(3)\"" w4807 {
                    tunnel: [_ u8[] [1, 2, 3, 4, 5, 6, 13, 8, 7, 9, 10, 11, 12] u8[] [1] u8[] [1] u8[] [2] u8[] [3] u8[] [4] u8[] [5] u8[] [6] u8[] [13] u8[] [7] u8[] [8] u8[] [9] u8[] [10] u8[] [14] u8[] [11] u8[] [12] u8[] [2] u8[] [3] u8[] [1] u8[] [2] u8[] [1] u8[] [2] u8[] [3] u8[] [4] u8[] [1, 2, 3, 4]] -> w4811
                    tunnel: [_ u8 128 ("命令") u8 129 ("命令") u8 128 ("命令") u8 128 ("命令") u8 128 ("命令") u8 128 ("命令") u8 128 ("命令") u8 128 ("命令") u8 128 ("命令") u8 128 ("命令") u8 128 ("命令") u8 128 ("命令") u8 128 ("命令") u8 128 ("命令") u8 128 ("命令") u8 128 ("命令") u8 129 ("命令") u8 129 ("命令") u8 130 ("命令") u8 130 ("命令") u8 132 ("命令") u8 132 ("命令") u8 132 ("命令") u8 132 ("命令") u8 132 ("命令")] -> w4810
                    tunnel: [_ string[] ["产品编号", "电压个数", "通道电压数", "电压起始值", "温度个数", "温度起始值", "保险位置", "电池额定实际容量", "SOC", "配置文件版本", "参数修改记录", "车牌号", "SOH"] string[] ["一级故障阀值"] string[] ["产品编号"] string[] ["电压个数"] string[] ["通道电压数"] string[] ["电压起始值"] string[] ["温度个数"] string[] ["温度起始值"] string[] ["保险位置"] string[] ["SOC"] string[] ["电池额定实际容量"] string[] ["配置文件版本"] string[] ["参数修改记录"] string[] ["校正时钟"] string[] ["车牌号"] string[] ["SOH"] string[] ["二级故障阀值"] string[] ["三级故障阀值"] string[] ["加热控制参数"] string[] ["充电控制参数"] string[] ["电池信息1"] string[] ["电池包组号"] string[] ["充放电安时"] string[] ["电池充放电次数"] string[] ["电池信息1", "电池包组号", "充放电安时", "电池充放电次数"]] -> w4806
                    frame "假", Default {
                    }
                    frame "项目信息" {
                    }
                    frame "SOC过低", "SOC过高", "SOH过低", "充电电流过高", "单体电压过低", "单体电压过高", "单组电压不均衡", "单组温度不均衡", "放电电流过高", "极柱温度过高", "内阻过大", "温度过低", "温度过高", "一级故障阀值", "整组电压不均衡", "整组温度不均衡", "总电压过低", "总电压过高" {
                    }
                    frame "产品编号" {
                    }
                    frame "电压个数" {
                    }
                    frame "通道电压数" {
                    }
                    frame "电压起始值" {
                    }
                    frame "温度个数" {
                    }
                    frame "温度起始值" {
                    }
                    frame "保险位置" {
                    }
                    frame "SOC" {
                    }
                    frame "电池额定实际容量" {
                    }
                    frame "配置文件版本" {
                    }
                    frame "参数修改记录" {
                    }
                    frame "校正时钟" {
                    }
                    frame "车牌号" {
                    }
                    frame "SOH" {
                    }
                    frame "SOC过低(2)", "SOC过高(2)", "SOH过低(2)", "充电电流过高(2)", "单体电压过低(2)", "单体电压过高(2)", "单组电压不均衡(2)", "单组温度不均衡(2)", "二级故障阀值", "放电电流过高(2)", "极柱温度过高(2)", "内阻过大(2)", "温度过低(2)", "温度过高(2)", "整组电压不均衡(2)", "整组温度不均衡(2)", "总电压过低(2)", "总电压过高(2)" {
                    }
                    frame "SOC过低(3)", "SOC过高(3)", "SOH过低(3)", "充电电流过高(3)", "单体电压过低(3)", "单体电压过高(3)", "单组电压不均衡(3)", "单组温度不均衡(3)", "放电电流过高(3)", "极柱温度过高(3)", "内阻过大(3)", "三级故障阀值", "温度过低(3)", "温度过高(3)", "整组电压不均衡(3)", "整组温度不均衡(3)", "总电压过低(3)", "总电压过高(3)" {
                    }
                    frame "风机关闭温差", "风机关闭温度", "风机开启温差", "风机开启温度", "加热关闭温差", "加热关闭温度", "加热开启温度", "加热控制参数" {
                    }
                    frame "充电控制参数", "电流步长", "最大允许充电电流", "最大允许充电温度", "最大允许单体电压", "最大允许总电压", "最小允许充电电流", "最小允许充电温度", "最小允许单体电压" {
                    }
                    frame "电池信息1" {
                    }
                    frame "电池包组号" {
                    }
                    frame "充放电安时" {
                    }
                    frame "电池充放电次数" {
                    }
                    frame "电池信息" {
                    }
                  }
                }
                frame "从板" {
                  n3497 = local read "从板选项"() -> (w4889:string)
                  n3498 = case shown="\"从板信息\"" w4889 {
                    tunnel: [_ u8 0 ("命令") u8 0 ("命令") u8 0 ("命令") u8 0 ("命令") u8 0 ("命令") u8 0 ("命令") u8 0 ("命令") u8 2 ("命令") u8 2 ("命令") u8 2 ("命令") u8 3 ("命令") u8 6 ("命令") u8 6 ("命令") u8 6 ("命令") u8 3 ("命令") u8 3 ("命令") u8 3 ("命令") u8 3 ("命令") u8 3 ("命令") u8 3 ("命令") u8 3 ("命令")] -> w4892
                    tunnel: [_ u8[] [6] u8[] [6, 1, 2, 3, 4, 5] u8[] [1] u8[] [2] u8[] [3] u8[] [4] u8[] [5] u8[] [1] u8[] [2] u8[] [3] u8[] [1, 2, 3, 4, 5, 6, 7] u8[] [1, 2] u8[] [2] u8[] [1] u8[] [1] u8[] [2] u8[] [3] u8[] [4] u8[] [5] u8[] [6] u8[] [7]] -> w4891
                    tunnel: [_ string[] ["从板号"] string[] ["从板号", "电压起始值", "通道电压个数", "保险位置", "温度起始值", "加热控制参数"] string[] ["电压起始值"] string[] ["通道电压节数"] string[] ["保险位置"] string[] ["温度起始值"] string[] ["加热控制参数"] string[] ["一级故障阀值"] string[] ["二级故障阀值"] string[] ["三级故障阀值"] string[] ["电池包信息1", "电池包序号", "充放电安时", "充电次数时间", "SOC", "车牌号", "充电参数"] string[] ["均衡阀值", "充电结束电压"] string[] ["充电结束电压"] string[] ["均衡阀值"] string[] ["电池包信息1"] string[] ["电池包序号"] string[] ["充放电安时"] string[] ["充电次数时间"] string[] ["SOC"] string[] ["车牌号"] string[] ["充电参数"]] -> w4887
                    frame "假", Default {
                    }
                    frame "从板号" {
                    }
                    frame "从板信息" {
                    }
                    frame "电压个数" {
                    }
                    frame "通道电压节数" {
                    }
                    frame "保险位置" {
                    }
                    frame "温度个数" {
                    }
                    frame "风机关闭温差", "风机关闭温度", "风机开启温差", "风机开启温度", "加热关闭温差", "加热关闭温度", "加热开启温度", "加热控制参数" {
                    }
                    frame "SOC过低", "电压不均衡", "电压过低", "电压过高", "温度不均衡", "温度过低", "温度过高", "一级故障阀值" {
                    }
                    frame "SOC过低(2)", "电压不均衡(2)", "电压过低(2)", "电压过高(2)", "二级故障阀值", "温度不均衡(2)", "温度过低(2)", "温度过高(2)" {
                    }
                    frame "SOC过低(3)", "电压不均衡(3)", "电压过低(3)", "电压过高(3)", "三级故障阀值", "温度不均衡(3)", "温度过低(3)", "温度过高(3)" {
                    }
                    frame "快换参数" {
                    }
                    frame "均衡参数" {
                    }
                    frame "充电结束电压" {
                    }
                    frame "均衡阀值" {
                    }
                    frame "电池包信息1" {
                    }
                    frame "电池包序号" {
                    }
                    frame "充放电安时" {
                    }
                    frame "充电次数时间" {
                    }
                    frame "SOC" {
                    }
                    frame "车牌号" {
                    }
                    frame "充电参数" {
                    }
                  }
                  n3499 = local read "从板号"() -> (w4888:u8)
                }
              }
              n3500 = Build Array(w4803) -> (w4802:i32[])
              n3501 = local write "命令"(w4805) -> ()
              n3502 = Array Size(array=w4800) -> (size(s)=w4799:i32)
              n3503 = for {
                tunnel: w4800 -> [w4964] mode=indexing
                tunnel: w4805 -> [w4963]
                tunnel: w4804 -> [w4962]
                tunnel: w4802 -> [w4961]
                tunnel: w4801 -> [w4960] mode=indexing
                tunnel: w4799 -> [w4959]
                tunnel: w4798 -> [w4957]
                tunnel: [w4956] -> w4797
                i -> [w4958]
                n3504 = while {
                  tunnel: w4964 -> [w4973]
                  tunnel: w4963 -> [w4972]
                  tunnel: w4962 -> [w4971]
                  tunnel: w4961 -> [w4970]
                  tunnel: w4960 -> [w4969]
                  tunnel: w4959 -> [w4968]
                  tunnel: w4958 -> [w4967]
                  tunnel: w4957 -> [w4966]
                  tunnel: [w4965] -> w4956
                  stop <- w4965 stop-if-true
                  n3505 = stacked-sequence {
                    seq-local: [_ _ _ _ w5121 _ _] -> [_ _ _ _ _ w5130 _]
                    tunnel: w4973 -> [_ _ _ w5109 _ _ _]
                    tunnel: w4972 -> [_ _ _ w5108 _ _ _]
                    tunnel: w4971 -> [_ _ _ w5107 _ _ _]
                    tunnel: w4970 -> [_ _ _ w5106 _ _ _]
                    tunnel: [_ _ _ _ w5122 _ _] -> w4965
                    tunnel: w4969 -> [w4975 _ _ _ _ w5131 _]
                    tunnel: w4968 -> [_ _ _ _ _ _ w5141]
                    tunnel: w4967 -> [_ _ _ _ _ _ w5140]
                    tunnel: w4966 -> [w4974 _ _ _ _ _ _]
                    frame #0 {
                      n3506 = case shown="\"主板\", 默认" w4974 {
                        tunnel: w4975 -> [w4976 w5067]
                        frame "主板", Default {
                          n3507 = case shown="\"电压个数\"" w4976 {
                            frame "假", Default {
                            }
                            frame "产品编号" {
                              n3508 = control-ref of="产品编号"() -> (w4978:refnum<vi>)
                              n3509 = property class="Str"(reference=w4978, "Value"="") -> ()  [unwired: 1 in, 2 out]
                            }
                            frame "电压个数" {
                              n3510 = local read "从板个数"() -> (w4979:dbl)
                              n3511 = control-ref of="项目信息"() -> (w4983:refnum<vi>)
                              n3512 = for {
                                N: w4979 -> [_]
                                tunnel: [""] -> w4982 mode=indexing
                              }
                              n3513 = call "表格数据输入-8.6.vi"("行数"=u32 0, "列数"=u32 1, "字符串数组"=w4982, "表格引用"=w4983) -> ()  [unwired: 8 in]
                            }
                            frame "通道电压数" {
                              n3514 = control-ref of="项目信息"() -> (w4989:refnum<vi>)
                              n3515 = for {
                                N: 20 -> [_]
                                tunnel: [""] -> w4988 mode=indexing
                              }
                              n3516 = local read "从板个数"() -> (w4990:dbl)
                              n3517 = Increment(x=w4990) -> (x+1=w4986:dbl)
                              n3518 = call "表格数据输入-8.6.vi"("行数"=w4986, "列数"=u32 1, "字符串数组"=w4988, "表格引用"=w4989) -> ()  [unwired: 8 in]
                            }
                            frame "电压起始值" {
                              n3519 = local read "从板个数"() -> (w4994:dbl)
                              n3520 = Increment(x=w4994) -> (x+1=w4993:dbl)
                              n3521 = control-ref of="项目信息"() -> (w5000:refnum<vi>)
                              n3522 = for {
                                N: w4993 -> [_]
                                tunnel: [""] -> w4999 mode=indexing
                              }
                              n3523 = Multiply(x=u8 1, y=w4994) -> (x*y=w4996:dbl)
                              n3524 = Add(x=w4996, y=u8 21) -> (x+y=w4992:dbl)
                              n3525 = call "表格数据输入-8.6.vi"("行数"=w4992, "列数"=u32 1, "字符串数组"=w4999, "表格引用"=w5000) -> ()  [unwired: 8 in]
                            }
                            frame "温度个数" {
                              n3526 = local read "从板个数"() -> (w5004:dbl)
                              n3527 = Increment(x=w5004) -> (x+1=w5003:dbl)
                              n3528 = control-ref of="项目信息"() -> (w5010:refnum<vi>)
                              n3529 = for {
                                N: w5003 -> [_]
                                tunnel: [""] -> w5009 mode=indexing
                              }
                              n3530 = Multiply(x=u8 2, y=w5004) -> (x*y=w5006:dbl)
                              n3531 = Add(x=w5006, y=u8 22) -> (x+y=w5002:dbl)
                              n3532 = call "表格数据输入-8.6.vi"("行数"=w5002, "列数"=u32 1, "字符串数组"=w5009, "表格引用"=w5010) -> ()  [unwired: 8 in]
                            }
                            frame "温度起始值" {
                              n3533 = local read "从板个数"() -> (w5014:dbl)
                              n3534 = Increment(x=w5014) -> (x+1=w5013:dbl)
                              n3535 = control-ref of="项目信息"() -> (w5020:refnum<vi>)
                              n3536 = for {
